vi "EncodeSingleCore.vi"(8 "error in (no error)":errorcluster, 10 "Data":string, 11 "Data Value Reference in":refnum<data-value>) -> (0 "error out":errorcluster, 3 "QR Code Image Data":u8[][](array[numeric]))   [LabVIEW 2020, in "feature_detection.lvlib" / "QR Code Encoder.lvclass"]
uses:
  QR Code Encoder.lvclass
  QR Code Encoder.lvclass/QR Code Encoder.ctl
  common/common.lvlib
  common/bin/gartoolkit_fd_32-1.dll
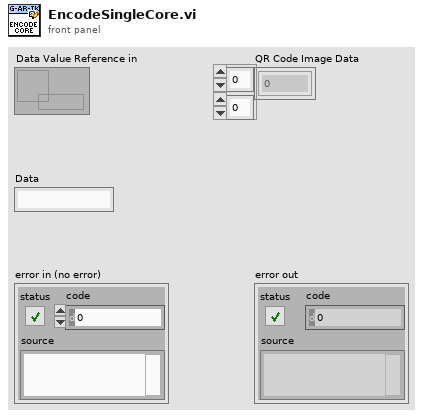
[diagram p1: front panel]
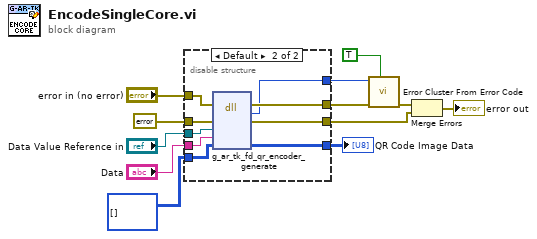
[diagram p0: block diagram]
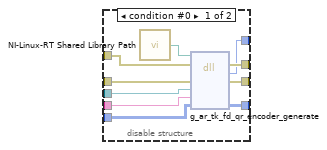
[diagram p2: hidden frame]
diagram:
  n1 = disable-structure "Conditional Disable Structure" shown="Default" {
    disable-tunnel: "error in (no error)" -> [w22 w31]
    disable-tunnel: errorcluster {"status"=FALSE, "code"=0, "source"=""} ("error constant") -> [w18 w30]
    disable-tunnel: [w21 w29] -> w4
    disable-tunnel: [w20 w28] -> w5
    disable-tunnel: [w17 w27] -> w6
    disable-tunnel: "Data Value Reference in" -> [w16 w26]
    disable-tunnel: "Data" -> [w15 w25]
    disable-tunnel: u8[][] [] -> [w14 w24]
    disable-tunnel: [w13 w23] -> w11
    frame condition #0 {
      n2 = call "NI-Linux-RT Shared Library Path.vi"() -> ("Path"=w19:path)
      n3 = dll-call lib="?" fn="g_ar_tk_fd_qr_encoder_generate" ("g_ar_toolkit.*.*:g_ar_tk_capture_context_create")(path in=w19, error in=w22, "error_cluster"=w18, "EDVR"=w16, "string"=w15, "output"=w14) -> (error out=w21:errorcluster, w20:i32, "error_cluster"=w17:errorcluster, "output"=w13:u8[][])  [unwired: 3 in, 1 out]
    }
    frame condition #1 (active) {
      n4 = dll-call lib="C:/serenial/lib/g-augmented-reality-toolkit/LabVIEW/common/bin/gartoolkit_fd_*-1.*" fn="g_ar_tk_fd_qr_encoder_generate" ("g_ar_toolkit.*.*:g_ar_tk_capture_context_create")(error in=w31, "error_cluster"=w30, "EDVR"=w26, "string"=w25, "output"=w24) -> (error out=w29:errorcluster, "return type"=w28:i32, "error_cluster"=w27:errorcluster, "output"=w23:u8[][])  [unwired: 4 in, 1 out]
    }
  }
  "QR Code Image Data" <- w11
  n5 = call <vilib>:"Error Cluster From Error Code.vi"("show call chain? (False)"=TRUE, "error in (no error)"=w4, "error code (0)"=w5) -> ("error out"=w2:errorcluster)  [unwired: 6 in]
  n6 = Merge Errors(w2, w6) -> (→"error out":errorcluster)
